vi "ReadGUIs.vi"(8 "Error In":errorcluster, 11 "object in":refnum<class "FrontPanelGUI.lvclass">) -> (0 "Error Out":errorcluster, 2 "GUIs":T2(array[cluster]), 3 "object out":refnum<class "FrontPanelGUI.lvclass">)   [LabVIEW 2021, in "TAF Proj Document Type.lvlib" / "FrontPanelGUI.lvclass"]
uses:
  <vilib>/Wovalab/AntiDoc/Document Type/Add-ons/LabVIEW TAF Project/FrontPanelGUI/FrontPanelGUI.lvclass
  <vilib>/picture/picture.llb/imagedata.ctl
  <vilib>/Wovalab/AntiDoc/Document Type/Add-ons/LabVIEW TAF Project/FrontPanelGUI/FrontPanelGUI.lvclass/FrontPanelGUI.ctl
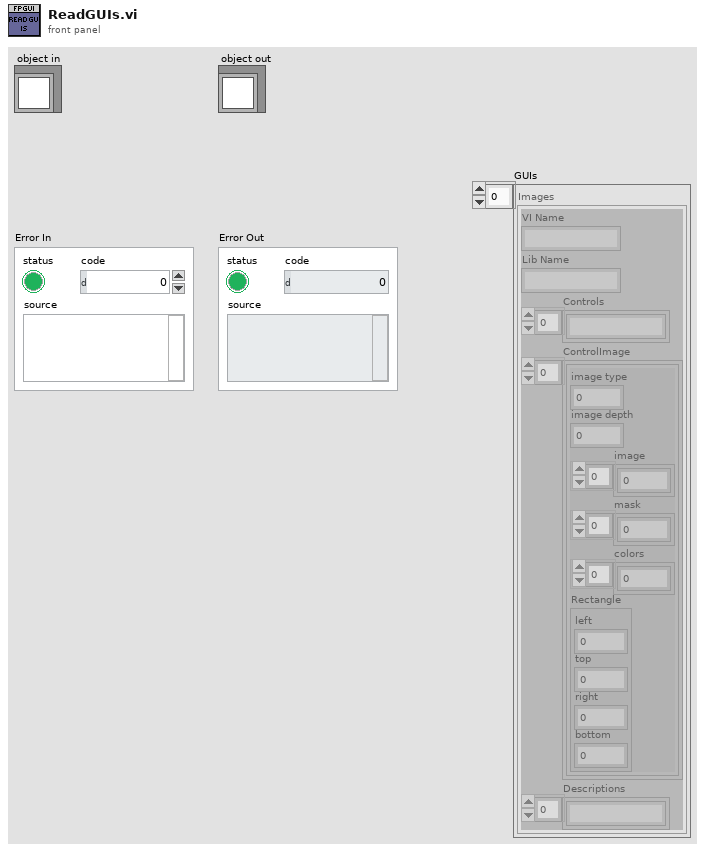
[diagram p1: front panel]
types:
  T1 = typedef "imagedata.ctl" = cluster{"image type":i32, "image depth":i32, "image":u8[], "mask":u8[], "colors":u32[], "Rectangle":cluster{"left":i16, "top":i16, "right":i16, "bottom":i16}}
  T2 = cluster{"VI Name":string, "Lib Name":string, "Controls":string[], "ControlImage":T1[], "Descriptions":string[]}[]
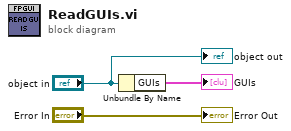
[diagram p0: block diagram]
diagram:
  n1 = Unbundle By Name("object in") -> ("GUIs"=→"GUIs":T2)
  "Error Out" <- "Error In"
  "object out" <- "object in"
